vi "Check Run Command Timer.vi"(10 "Timeout (ms)":u32=5000, 11 "CIF_UI in":refnum<class "CIF_UI.lvclass">) -> (3 "Timeout":bool)   [LabVIEW 2021, in "CIF_UI.lvclass"]
uses:
  CIF_UI.lvclass
  CIF_UI.lvclass/CIF_UI.ctl
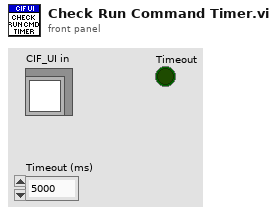
[diagram p1: front panel]
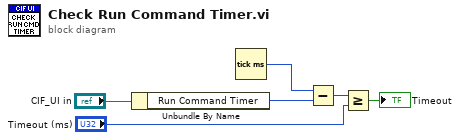
[diagram p0: block diagram]
diagram:
  n1 = Unbundle By Name("CIF_UI in") -> ("Run Command Timer"=w3:u32)
  n2 = Tick Count (ms)() -> (millisecond timer value=w2:u32)
  n3 = Subtract(x=w2, y=w3) -> (x-y=w1:u32)
  n4 = Greater Or Equal?(x=w1, y="Timeout (ms)") -> (x >= y?=→"Timeout":bool)
